vi "Get Shared Registers.vi"(2 "shared":refnum<class "niUSRP Rx Core v1 FPGA.lvclass">=refnum) -> (4 "shared registers":refnum<class "Address Space Collection.lvclass">)   [LabVIEW 2023]
uses:
  <instrlib>/_niInstr/Instruction Framework/v1/FPGA/Interfaces/Address Space Collection/Address Space Collection.lvclass
  <instrlib>/niUSRP/Reference FPGA/Rx Core/niUSRP Rx Core v1 FPGA.lvclass
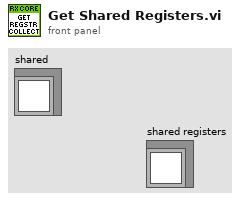
[diagram p1: front panel]
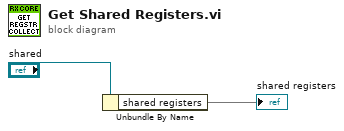
[diagram p0: block diagram]
diagram:
  n1 = Unbundle By Name("shared") -> ("shared registers"=→"shared registers")
